vi "Format String.vi"(10 "String":string) -> (2 "Formatted String":string)   [LabVIEW 2016, in "Stream Log.lvlib" / "Text File Sink.lvclass"]
doc: "--\nCopyright © 2017 Composed SystemsI All rights reserved.\n\nAuthor: Jon McBee <jon.mcbee@composed.io>\n\nThis library is provided \"AS IS\" ,WITHOUT WARRANTIES OR\nCONDITIONS OF ANY KIND, either express or implied.\n\nComposed Systems -- composed.io\n\nStream 0.0.1.1\nJon McBee - Composed Systems\nCopyright (c) 2017, Composed Systems"
uses:
  <userlib>/Composed Systems/Stream/Log/Text File Sink/Text File Sink.lvclass
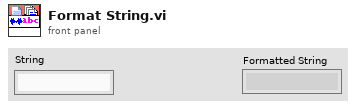
[diagram p1: front panel]
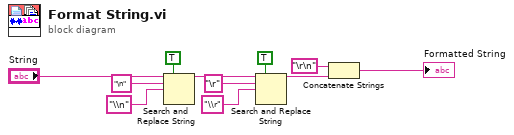
[diagram p0: block diagram]
diagram:
  n1 = Search and Replace String(replace all?=TRUE ("replace all? (F)"), input string="String", search string="\n", replace string="\\n" ("replace string (\"\")")) -> (result string=w3:string)  [unwired: 1 in, 6 out]
  n2 = Search and Replace String(replace all?=TRUE ("replace all? (F)"), input string=w3, search string="\r", replace string="\\r" ("replace string (\"\")")) -> (result string=w2:string)  [unwired: 1 in, 6 out]
  n3 = Concatenate Strings("\r\n", w2) -> (→"Formatted String":string)
